vi "Replace.vi"(1 "data in":u8[][][](array[numeric]), 2 "threshold":dbl format="%.2f") -> (0 "data out":u8[][][](array[numeric]))   [LabVIEW 2022 SP3]
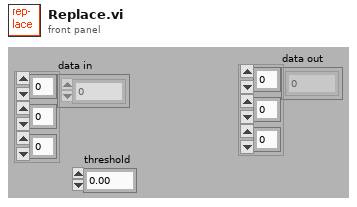
[diagram p1: front panel]
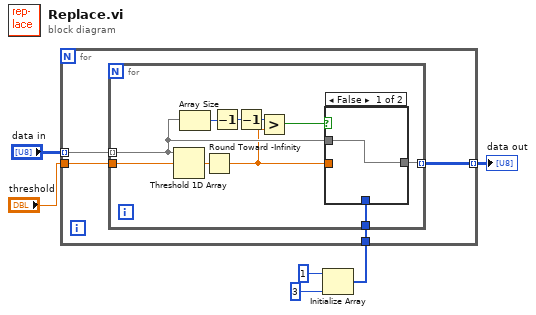
[diagram p0: block diagram]
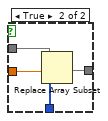
[diagram p2: hidden frame]
diagram:
  n1 = Initialize Array(1, 3) -> (w2:i32[])
  n2 = for {
    tunnel: "threshold" -> [w10]
    tunnel: "data in" -> [w9] mode=indexing
    tunnel: [w8] -> w4 mode=indexing
    tunnel: w2 -> [w7]
    n3 = for {
      tunnel: w10 -> [w20]
      tunnel: w9 -> [w16] mode=indexing
      tunnel: [w18] -> w8 mode=indexing
      tunnel: w7 -> [w17]
      n4 = Threshold 1D Array(2:w20, 3:w16) -> (0:w19:dbl)  [unwired: 1 out]
      n5 = Array Size(array=w16) -> (size(s)=w15:i32)
      n6 = Round Toward -Infinity(1:w19) -> (0:w13:dbl)
      n7 = Decrement(x=w15) -> (x-1=w14:i32)
      n8 = Decrement(x=w14) -> (x-1=w12:i32)
      n9 = Greater?(x=w12, y=w13) -> (0:w11:bool)
      n10 = case shown="False" w11 {
        tunnel: [w21 w25] -> w18
        tunnel: w17 -> [_ w24]
        tunnel: w16 -> [w21 w23]
        tunnel: w13 -> [_ w22]
        frame False {
        }
        frame True {
          n11 = Replace Array Subset(array=w23, new element=w24, index=w22) -> (w25:u8[])
        }
      }
    }
  }
  "data out" <- w4
